vi "Dev Mode Hide.vi"(7 "Developer Mode?":bool, 8 "error in (no error)":errorcluster, 11 "Pages":refnum<vi>[](array[refnum])) -> (0 "error out":errorcluster)   [LabVIEW 2020]
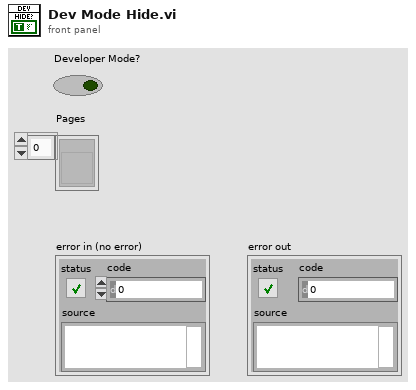
[diagram p1: front panel]
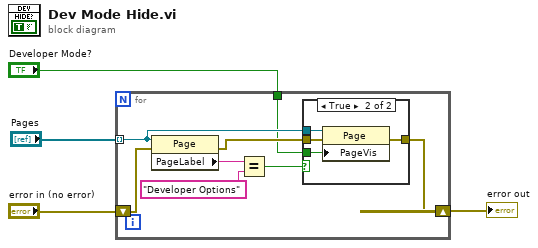
[diagram p0: block diagram]
diagram:
  n1 = for {
    tunnel: "Pages" -> [w10] mode=indexing
    shift-right: [w7] -> w4
    shift-left: "error in (no error)" -> [w9]
    tunnel: "Developer Mode?" -> [w6]
    n2 = property class="Page"(reference=w10, error in=w9) -> (error out=w8:errorcluster, "PageLabel"=w12:string)  [unwired: 1 out]
    n3 = Equal?(x=w12, y="Developer Options") -> (x = y?=w5:bool)
    n4 = case shown="True" w5 {
      tunnel: w10 -> [_ w17]
      tunnel: w8 -> [w13 w16]
      tunnel: [w13 w15] -> w7
      tunnel: w6 -> [_ w14]
      frame False {
      }
      frame True {
        n5 = property class="Page"(reference=w17, error in=w16, "PageVis"=w14) -> (error out=w15:errorcluster)  [unwired: 1 out]
      }
    }
  }
  "error out" <- w4
